vi "specu1a 1.0.0 Read SYS version.vi"(3 "error in (no error)":errorcluster, 5 "Device Handle":i32) -> (0 "error out":errorcluster, 1 "SYS Version":string, 2 "Device Handle out":i32)   [LabVIEW 2010]
uses:
  WINDOWS/SYSTEM32/DRIVERS/specu1a.dll
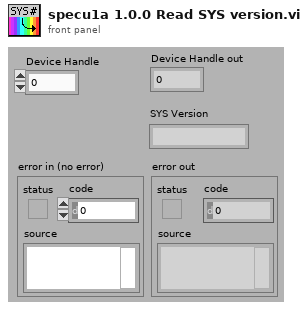
[diagram p1: front panel]
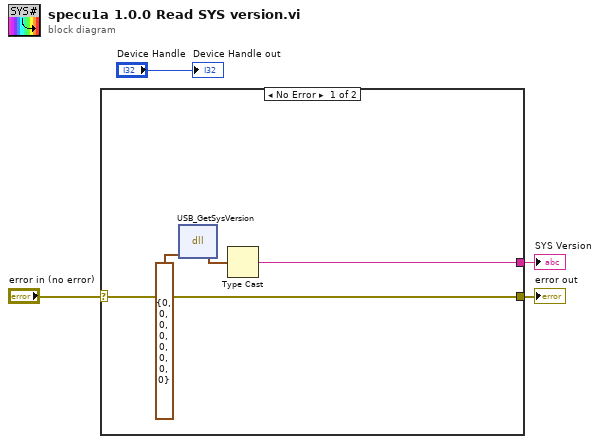
[diagram p0: block diagram]
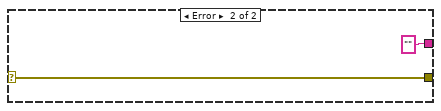
[diagram p2: hidden frame]
diagram:
  n1 = case shown="No Error" "error in (no error)" {
    selector: "error in (no error)" -> [w7 w10]
    tunnel: [w7 w10] -> w3
    tunnel: [w8 ""] -> w1
    frame No Error {
      n2 = dll-call lib="C:/SpecUSB Drivers/DLL&Driver/specu1a.dll" fn="USB_GetSysVersion" label="1.0.0 Get SYS Version"(cluster{u8, u8, u8, u8, u8, u8, u8, u8} {0, 0, 0, 0, 0, 0, 0, 0}) -> (w5:cluster{u8, u8, u8, u8, u8, u8, u8, u8})  [unwired: 4 in, 2 out]
      n3 = Type Cast(x=w5) -> (*(type *) &x=w8:string)  [unwired: 1 in]
    }
    frame Error {
    }
  }
  "error out" <- w3
  "SYS Version" <- w1
  "Device Handle out" <- "Device Handle"
